vi "LWXPS_GPIODigitalGet.vi"(0 "XPS Reference IN":refnum<k24>, 5 "GPIO Name":string, 11 "LabVIEW error IN":errorcluster) -> (4 "XPS Reference OUT":refnum<k24>, 6 "Returned error code":i32, 8 "Digital Value":u16, 10 "XPS Error String":string, 15 "LabVIEW error OUT":errorcluster)   [LabVIEW 2014]
uses:
  D:/XPSQ8_LabView_Library/Development/Source/Dll/Newport.XPS.CommandInterface.dll
  Dll/Newport.XPS.CommandInterface.dll
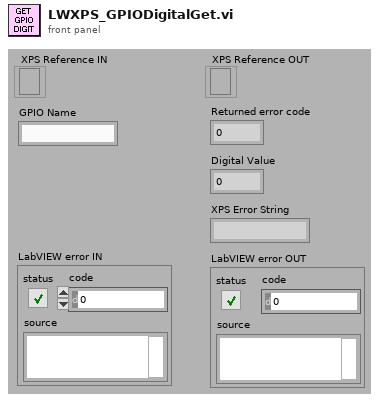
[diagram p1: front panel]
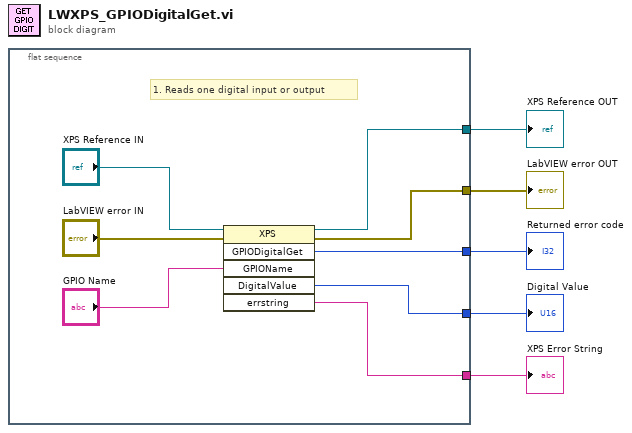
[diagram p0: block diagram]
diagram:
  n1 = flat-sequence {
    tunnel: [w10] -> w5
    tunnel: [w13] -> w4
    tunnel: [w11] -> w3
    tunnel: [w9] -> w1
    tunnel: [w8] -> w2
    frame #0 {
      # "1. Reads one digital input or output"
      n2 = invoke class="XPS" method="GPIODigitalGet"(reference="XPS Reference IN", error in="LabVIEW error IN", "GPIOName"="GPIO Name") -> (reference out=w10:refnum<k24>, error out=w13:errorcluster, "GPIODigitalGet"=w11:i32, "DigitalValue"=w9:u16, "errstring"=w8:string)  [unwired: 3 in, 1 out]
    }
  }
  "XPS Reference OUT" <- w5
  "LabVIEW error OUT" <- w4
  "Returned error code" <- w3
  "XPS Error String" <- w2
  "Digital Value" <- w1
